vi "Get IDs.vi"(11 "Linked List Definition in":refnum<class "Linked List Definition.lvclass">) -> (1 "Data IDs":string[](array[string]), 3 "Child IDs":string[](array[string]), 4 "Linked List ID":string)   [LabVIEW 2019, in "Linked Lists.lvlib" / "Linked List Definition.lvclass"]
uses:
  <vilib>/gpm_packages/@cs/linked-list/Source/Linked List/Linked List Definition/Linked List Definition.lvclass
  <vilib>/gpm_packages/@cs/linked-list/Source/Linked List/Linked List Definition/Linked List Definition.lvclass/Linked List Definition.ctl
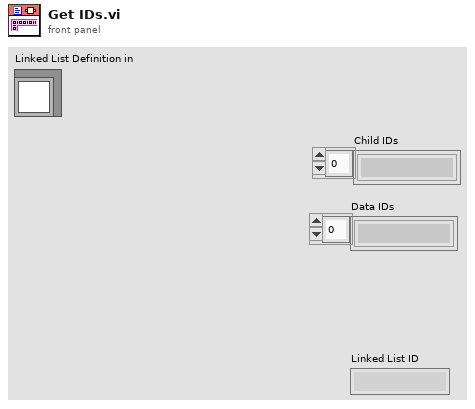
[diagram p1: front panel]
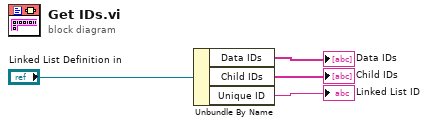
[diagram p0: block diagram]
diagram:
  n1 = Unbundle By Name("Linked List Definition in") -> ("Data IDs"=→"Data IDs":string[], "Child IDs"=→"Child IDs":string[], "Unique ID"=→"Linked List ID":string)
